vi "errorUDP.vi"(8 "error in (no error) 2":errorcluster, 11 "errorcode":i32=60) -> (0 "error out 2":errorcluster)   [LabVIEW 2014]
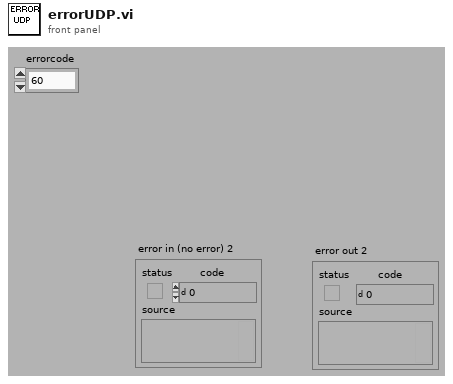
[diagram p1: front panel]
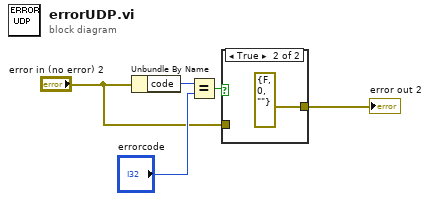
[diagram p0: block diagram]
diagram:
  n1 = Unbundle By Name("error in (no error) 2") -> ("code"=w5:i32)
  n2 = Equal?(x=w5, y="errorcode") -> (x = y?=w3:bool)
  n3 = case shown="True" w3 {
    tunnel: "error in (no error) 2" -> [w6 _]
    tunnel: [w6 errorcluster {"status"=FALSE, "code"=0, "source"=""} ("error out")] -> w1
    frame False {
    }
    frame True {
    }
  }
  "error out 2" <- w1
